vi "PCSMain.get System Objects.vi"(1 "DB Entries":cluster{"Object Name":string, "Class":string}[](array[cluster])) -> (0 "Many i attributes":T1={"System Objects"={"Spectrometer Objects"=[], "Camera Objects"=[], "Image Operator Objects"=[], "Gate- and Delaygenerators"=[], "Current Meas Objects"=[], "Calorimeter Objects"=[], "Powermeter Objects"=[], "SSAC Objects"=[], "Vacuum Control Objects"=[], "Countdown Counter Objects"=[], "Beckhoff Watchdog Objects"=[], "SHS Analyzer Objects"=[]}, "Local Objects"={"Spectrometer Objects"=[], "Camera Objects"=[], "Image Operator Objects"=[], "Gate- and Delaygenerators"=[], "Current Meas Objects"=[], "Calorimeter Objects"=[], "Powermeter Objects"=[], "SSAC Objects"=[], "Vacuum Control Objects"=[], "Countdown Counter Objects"=[], "Beckhoff Watchdog Objects"=[], "SHS Analyzer Objects"=[]}, "Systems on same node"=[], "Data Viewer visible?"=FALSE, "Running Objects"={"Operators"=FALSE, "SHS Analyzers"=FALSE}, "Cam Instance System ID"="N/A", "Black Box Objects"=[], "Switch Objects"=[], "Motion GUI Objects"=[], "Osci Objects"=[]})   [LabVIEW 2014, in "PCSMain.lvlib"]
doc: "This VI requires the data base entries as an array of clusters which consists of the object names and class and writes them to own attributes."
uses:
  PCSMain.lvlib
  PCSMain.i attribute.ctl
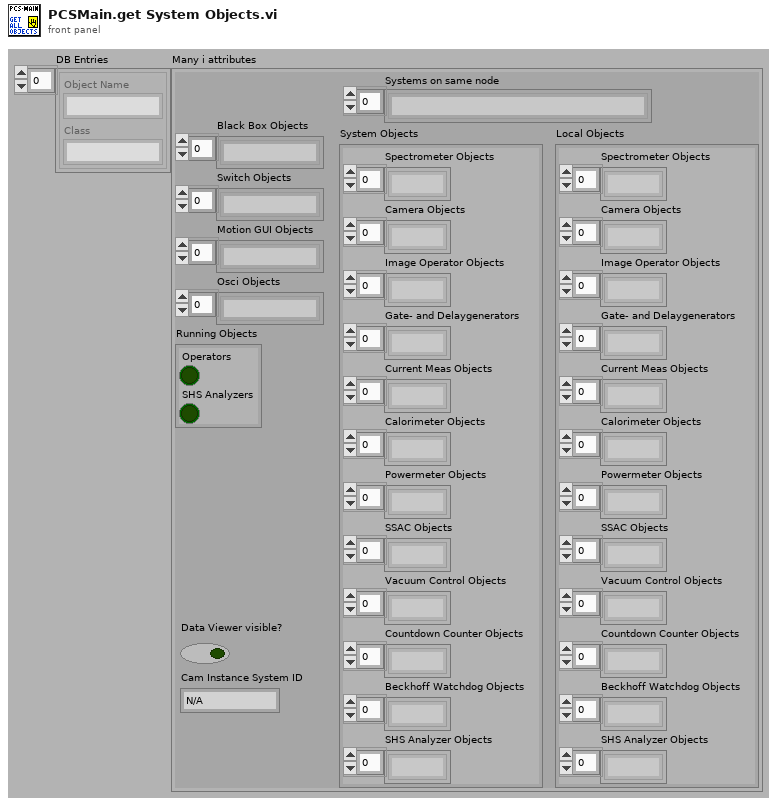
[diagram p1: front panel]
types:
  T1 = typedef "PCSMain.lvlib/PCSMain.i attribute.ctl" = cluster{"System Objects":cluster{"Spectrometer Objects":string[], "Camera Objects":string[], "Image Operator Objects":string[], "Gate- and Delaygenerators":string[], "Current Meas Objects":string[], "Calorimeter Objects":string[], "Powermeter Objects":string[], "SSAC Objects":string[], "Vacuum Control Objects":string[], "Countdown Counter Objects":string[], "Beckhoff Watchdog Objects":string[], "SHS Analyzer Objects":string[]}, "Local Objects":cluster{"Spectrometer Objects":string[], "Camera Objects":string[], "Image Operator Objects":string[], "Gate- and Delaygenerators":string[], "Current Meas Objects":string[], "Calorimeter Objects":string[], "Powermeter Objects":string[], "SSAC Objects":string[], "Vacuum Control Objects":string[], "Countdown Counter Objects":string[], "Beckhoff Watchdog Objects":string[], "SHS Analyzer Objects":string[]}, "Systems on same node":string[], "Data Viewer visible?":bool, "Running Objects":cluster{"Operators":bool, "SHS Analyzers":bool}, "Cam Instance System ID":string, "Black Box Objects":string[], "Switch Objects":string[], "Motion GUI Objects":string[], "Osci Objects":string[]}
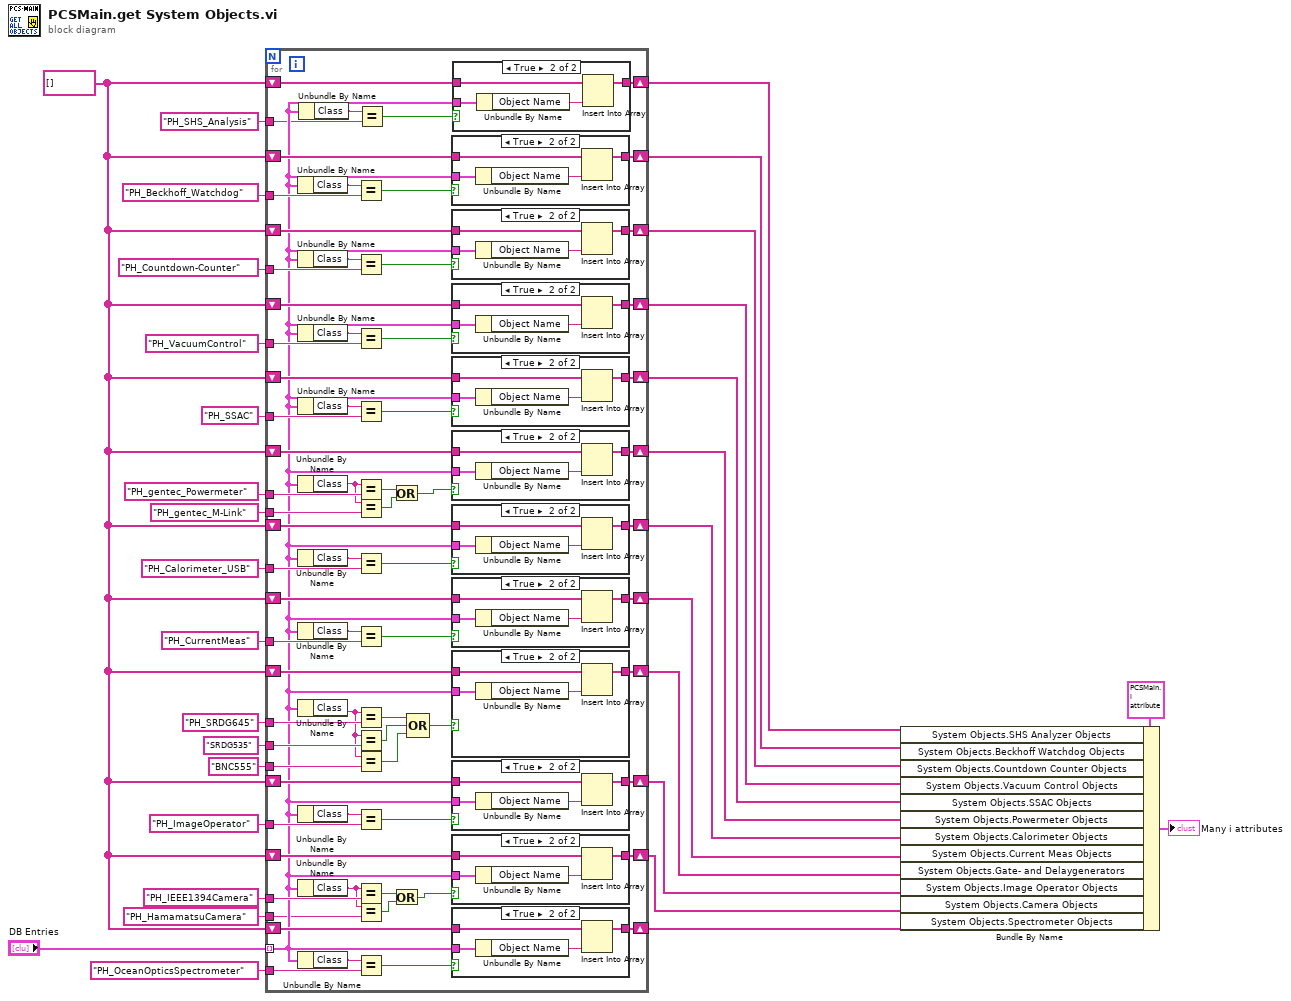
[diagram p0: block diagram]
diagram:
  w6 = string[] [] ("DB - Local Objects to open.Spectrometer Objects")
  n1 = for {
    tunnel: "PH_OceanOpticsSpectrometer" ("Class") -> [w104]
    tunnel: "DB Entries" -> [w39] mode=indexing
    shift-right: [w101] -> w30
    shift-left: w6 -> [w100]
    shift-right: [w98] -> w29
    shift-left: w6 -> [w99]
    tunnel: "PH_IEEE1394Camera" ("Class") -> [w97]
    shift-right: [w94] -> w26
    shift-left: w6 -> [w93]
    tunnel: "PH_ImageOperator" ("Class") -> [w92]
    shift-right: [w50] -> w25
    shift-left: w6 -> [w51]
    shift-right: [w87] -> w24
    shift-left: w6 -> [w85]
    shift-right: [w86] -> w23
    shift-left: w6 -> [w84]
    tunnel: "PH_Calorimeter_USB" -> [w83]
    tunnel: "PH_CurrentMeas" -> [w82]
    tunnel: "SRDG535" -> [w57]
    tunnel: "BNC555" -> [w81]
    shift-right: [w80] -> w17
    shift-left: w6 -> [w79]
    tunnel: "PH_gentec_Powermeter" -> [w78]
    tunnel: "PH_SSAC" ("Class") -> [w75]
    shift-right: [w73] -> w15
    shift-left: w6 -> [w74]
    shift-right: [w72] -> w14
    shift-left: w6 -> [w71]
    tunnel: "PH_VacuumControl" ("Class") -> [w68]
    shift-right: [w67] -> w11
    shift-left: w6 -> [w66]
    tunnel: "PH_Countdown-Counter" ("Class") -> [w64]
    shift-right: [w59] -> w9
    shift-left: w6 -> [w60]
    tunnel: "PH_Beckhoff_Watchdog" ("Class") -> [w58]
    tunnel: "PH_SRDG645" -> [w55]
    tunnel: "PH_gentec_M-Link" -> [w48]
    shift-right: [w43] -> w4
    shift-left: w6 -> [w42]
    tunnel: "PH_SHS_Analysis" -> [w38]
    tunnel: "PH_HamamatsuCamera" ("Class") -> [w36]
    n2 = Unbundle By Name(w39) -> ("Class"=w62:string)
    n3 = Unbundle By Name(w39) -> ("Class"=w65:string)
    n4 = Unbundle By Name(w39) -> ("Class"=w70:string)
    n5 = Unbundle By Name(w39) -> ("Class"=w77:string)
    n6 = Unbundle By Name(w39) -> ("Class"=w47:string)
    n7 = Unbundle By Name(w39) -> ("Class"=w88:string)
    n8 = Unbundle By Name(w39) -> ("Class"=w90:string)
    n9 = Unbundle By Name(w39) -> ("Class"=w54:string)
    n10 = Unbundle By Name(w39) -> ("Class"=w95:string)
    n11 = Unbundle By Name(w39) -> ("Class"=w37:string)
    n12 = Unbundle By Name(w39) -> ("Class"=w102:string)
    n13 = Unbundle By Name(w39) -> ("Class"=w41:string)
    n14 = Equal?(x=w62, y=w58) -> (x = y?=w61:bool)
    n15 = Equal?(x=w65, y=w64) -> (x = y?=w63:bool)
    n16 = Equal?(x=w70, y=w68) -> (x = y?=w69:bool)
    n17 = Equal?(x=w77, y=w75) -> (x = y?=w76:bool)
    n18 = Equal?(x=w47, y=w78) -> (x = y?=w45:bool)
    n19 = Equal?(x=w47, y=w48) -> (x = y?=w44:bool)
    n20 = Equal?(x=w88, y=w83) -> (x = y?=w89:bool)
    n21 = Equal?(x=w90, y=w82) -> (x = y?=w91:bool)
    n22 = Equal?(x=w54, y=w55) -> (x = y?=w53:bool)
    n23 = Equal?(x=w54, y=w57) -> (x = y?=w56:bool)
    n24 = Equal?(x=w54, y=w81) -> (x = y?=w52:bool)
    n25 = Equal?(x=w95, y=w92) -> (x = y?=w96:bool)
    n26 = Equal?(x=w37, y=w97) -> (x = y?=w34:bool)
    n27 = Equal?(x=w37, y=w36) -> (x = y?=w35:bool)
    n28 = Equal?(x=w102, y=w104) -> (x = y?=w103:bool)
    n29 = Equal?(x=w41, y=w38) -> (x = y?=w40:bool)
    n30 = Or(x=w45, y=w44) -> (x .or. y?=w46:bool)
    n31 = Or(x=w34, y=w35) -> (x .or. y?=w33:bool)
    n32 = Compound Arithmetic op=OR(w53, w56, w52) -> (w49:bool)
    n33 = case shown="True" w61 {
      tunnel: w39 -> [_ w117]
      tunnel: [w115 w119] -> w59
      tunnel: w60 -> [w115 w118]
      frame False {
      }
      frame True {
        n34 = Unbundle By Name(w117) -> ("Object Name"=w116:string)
        n35 = Insert Into Array(array=w118, new element=w116) -> (w119:string[])  [unwired: 1 in]
      }
    }
    n36 = case shown="True" w63 {
      tunnel: w39 -> [_ w122]
      tunnel: [w120 w124] -> w67
      tunnel: w66 -> [w120 w123]
      frame False {
      }
      frame True {
        n37 = Unbundle By Name(w122) -> ("Object Name"=w121:string)
        n38 = Insert Into Array(array=w123, new element=w121) -> (w124:string[])  [unwired: 1 in]
      }
    }
    n39 = case shown="True" w69 {
      tunnel: w39 -> [_ w127]
      tunnel: [w125 w129] -> w72
      tunnel: w71 -> [w125 w128]
      frame False {
      }
      frame True {
        n40 = Unbundle By Name(w127) -> ("Object Name"=w126:string)
        n41 = Insert Into Array(array=w128, new element=w126) -> (w129:string[])  [unwired: 1 in]
      }
    }
    n42 = case shown="True" w76 {
      tunnel: w39 -> [_ w132]
      tunnel: [w130 w134] -> w73
      tunnel: w74 -> [w130 w133]
      frame False {
      }
      frame True {
        n43 = Unbundle By Name(w132) -> ("Object Name"=w131:string)
        n44 = Insert Into Array(array=w133, new element=w131) -> (w134:string[])  [unwired: 1 in]
      }
    }
    n45 = case shown="True" w46 {
      tunnel: [w135 w139] -> w80
      tunnel: w79 -> [w135 w137]
      tunnel: w39 -> [_ w136]
      frame False {
      }
      frame True {
        n46 = Unbundle By Name(w136) -> ("Object Name"=w138:string)
        n47 = Insert Into Array(array=w137, new element=w138) -> (w139:string[])  [unwired: 1 in]
      }
    }
    n48 = case shown="True" w89 {
      tunnel: [w140 w144] -> w86
      tunnel: w84 -> [w140 w142]
      tunnel: w39 -> [_ w141]
      frame False {
      }
      frame True {
        n49 = Unbundle By Name(w141) -> ("Object Name"=w143:string)
        n50 = Insert Into Array(array=w142, new element=w143) -> (w144:string[])  [unwired: 1 in]
      }
    }
    n51 = case shown="True" w91 {
      tunnel: [w145 w149] -> w87
      tunnel: w85 -> [w145 w147]
      tunnel: w39 -> [_ w146]
      frame False {
      }
      frame True {
        n52 = Unbundle By Name(w146) -> ("Object Name"=w148:string)
        n53 = Insert Into Array(array=w147, new element=w148) -> (w149:string[])  [unwired: 1 in]
      }
    }
    n54 = case shown="True" w49 {
      tunnel: [w110 w114] -> w50
      tunnel: w51 -> [w110 w112]
      tunnel: w39 -> [_ w111]
      frame False {
      }
      frame True {
        n55 = Unbundle By Name(w111) -> ("Object Name"=w113:string)
        n56 = Insert Into Array(array=w112, new element=w113) -> (w114:string[])  [unwired: 1 in]
      }
    }
    n57 = case shown="True" w96 {
      tunnel: [w150 w154] -> w94
      tunnel: w93 -> [w150 w152]
      tunnel: w39 -> [_ w151]
      frame False {
      }
      frame True {
        n58 = Unbundle By Name(w151) -> ("Object Name"=w153:string)
        n59 = Insert Into Array(array=w152, new element=w153) -> (w154:string[])  [unwired: 1 in]
      }
    }
    n60 = case shown="True" w33 {
      tunnel: w39 -> [_ w158]
      tunnel: [w155 w159] -> w98
      tunnel: w99 -> [w155 w156]
      frame False {
      }
      frame True {
        n61 = Unbundle By Name(w158) -> ("Object Name"=w157:string)
        n62 = Insert Into Array(array=w156, new element=w157) -> (w159:string[])  [unwired: 1 in]
      }
    }
    n63 = case shown="True" w103 {
      tunnel: w39 -> [_ w162]
      tunnel: [w160 w164] -> w101
      tunnel: w100 -> [w160 w163]
      frame False {
      }
      frame True {
        n64 = Unbundle By Name(w162) -> ("Object Name"=w161:string)
        n65 = Insert Into Array(array=w163, new element=w161) -> (w164:string[])  [unwired: 1 in]
      }
    }
    n66 = case shown="True" w40 {
      tunnel: w39 -> [_ w107]
      tunnel: [w105 w109] -> w43
      tunnel: w42 -> [w105 w108]
      frame False {
      }
      frame True {
        n67 = Unbundle By Name(w107) -> ("Object Name"=w106:string)
        n68 = Insert Into Array(array=w108, new element=w106) -> (w109:string[])  [unwired: 1 in]
      }
    }
  }
  n69 = Bundle By Name(cluster=T1 {"System Objects"={"Spectrometer Objects"=[], "Camera Objects"=[], "Image Operator Objects"=[], "Gate- and Delaygenerators"=[], "Current Meas Objects"=[], "Calorimeter Objects"=[], "Powermeter Objects"=[], "SSAC Objects"=[], "Vacuum Control Objects"=[], "Countdown Counter Objects"=[], "Beckhoff Watchdog Objects"=[], "SHS Analyzer Objects"=[]}, "Local Objects"={"Spectrometer Objects"=[], "Camera Objects"=[], "Image Operator Objects"=[], "Gate- and Delaygenerators"=[], "Current Meas Objects"=[], "Calorimeter Objects"=[], "Powermeter Objects"=[], "SSAC Objects"=[], "Vacuum Control Objects"=[], "Countdown Counter Objects"=[], "Beckhoff Watchdog Objects"=[], "SHS Analyzer Objects"=[]}, "Systems on same node"=[], "Data Viewer visible?"=FALSE, "Running Objects"={"Operators"=FALSE, "SHS Analyzers"=FALSE}, "Cam Instance System ID"="", "Black Box Objects"=[], "Switch Objects"=[], "Motion GUI Objects"=[], "Osci Objects"=[]} ("CLASS.i attribute"), "System Objects.SHS Analyzer Objects"=w4, "System Objects.Beckhoff Watchdog Objects"=w9, "System Objects.Countdown Counter Objects"=w11, "System Objects.Vacuum Control Objects"=w14, "System Objects.SSAC Objects"=w15, "System Objects.Powermeter Objects"=w17, "System Objects.Calorimeter Objects"=w23, "System Objects.Current Meas Objects"=w24, "System Objects.Gate- and Delaygenerators"=w25, "System Objects.Image Operator Objects"=w26, "System Objects.Camera Objects"=w29, "System Objects.Spectrometer Objects"=w30) -> (→"Many i attributes":T1)
